vi "Next Turn.vi"(8 "error in (no error)":errorcluster, 11 "Reversi in":refnum<class "Reversi.lvclass">) -> (0 "error out":errorcluster, 3 "Reversi out":refnum<class "Reversi.lvclass">)   [LabVIEW 2020, in "Reversi.lvlib" / "Reversi.lvclass"]
uses:
  Reversi.lvclass
  Reversi.lvclass/Reversi.ctl
  Turn Enum.ctl
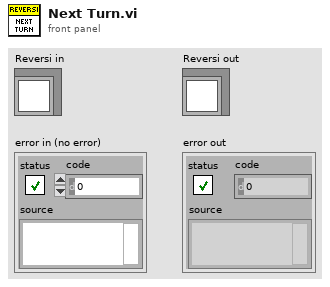
[diagram p1: front panel]
types:
  T1 = typedef "Reversi.lvlib/Reversi.lvclass/Turn Enum.ctl" = enum16{"Black", "White"}
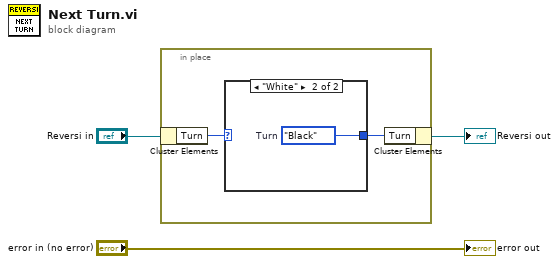
[diagram p0: block diagram]
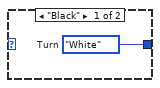
[diagram p2: hidden frame]
diagram:
  n1 = in-place {
    n2 = in-place-cluster #1("Reversi in") -> ("Turn"=w5:T1)
    n3 = case shown="\"White\"" w5 {
      tunnel: [w6 w7] -> w4
      frame "Black" {
        w6 = Turn_Enum."White"  # Turn
      }
      frame "White" {
        w7 = Turn_Enum."Black"  # Turn
      }
    }
    n4 = in-place-cluster #1("Turn"=w4) -> (→"Reversi out":refnum<class "Reversi.lvclass">)
  }
  "error out" <- "error in (no error)"
